vi "Close.vi"(8 "Error In":errorcluster, 11 "SFTP File":refnum<class "SFTP File.lvclass">) -> (0 "Error Out":errorcluster, 2 "Remote Path":string, 3 "SFTP":refnum<class "SFTP.lvclass">)   [LabVIEW 2018, in "Toolkit.lvlib" / "SFTP File.lvclass"]
uses:
  SFTP File.lvclass
  SFTP/SFTP.lvclass
  SFTP File.lvclass/SFTP File.ctl
  SFTP/SFTP.lvclass/SFTP.ctl
  Toolkit.lvlib
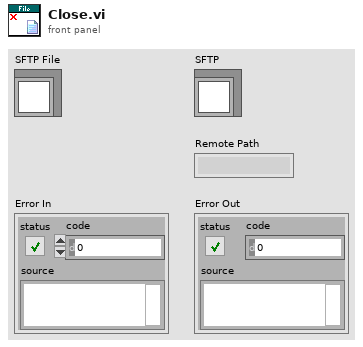
[diagram p1: front panel]
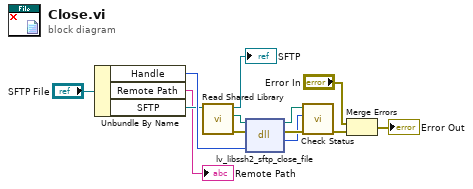
[diagram p0: block diagram]
diagram:
  n1 = Unbundle By Name("SFTP File") -> ("Handle"=w11:u64, "Remote Path"=→"Remote Path":string, "SFTP"=w5:refnum<class "SFTP.lvclass">)
  n2 = call "Read Shared Library.vi"("SFTP In"=w5) -> ("Erorr Out"=w2:errorcluster, "lv-libssh2 Shared Library"=w3:path, "SFTP Out"=→"SFTP":refnum<class "SFTP.lvclass">)  [unwired: 8 in]
  n3 = dll-call lib="D:/Users/cfield/Code/Field R&D Services/SSH/LV-LIBSSH2/LabVIEW/trunk/src/Toolkit/Support/lv-libssh2.dll" fn="lv_libssh2_sftp_close_file"(path in=w3, error in=w2, "handle"=w11) -> (path out=w9:path, error out=w10:errorcluster, "status"=w7:i32)  [unwired: 2 in]
  n4 = call "Check Status.vi"("Error In"=w10, "Status"=w7, "lv-libssh2 Shared Library In"=w9) -> ("Error Out"=w8:errorcluster)  [unwired: 7 in, 1 out]
  n5 = Merge Errors("Error In", w8) -> (→"Error Out":errorcluster)
